vi "Close.vi"(8 "error in (no error)":errorcluster, 11 "SolarShutt in":refnum<class "SolarShutt.lvclass">) -> (0 "error out":errorcluster, 3 "SolarShutt out":refnum<class "SolarShutt.lvclass">)   [LabVIEW 2016]
uses:
  SolarShutt.lvclass
  Controls/Shutter States.ctl
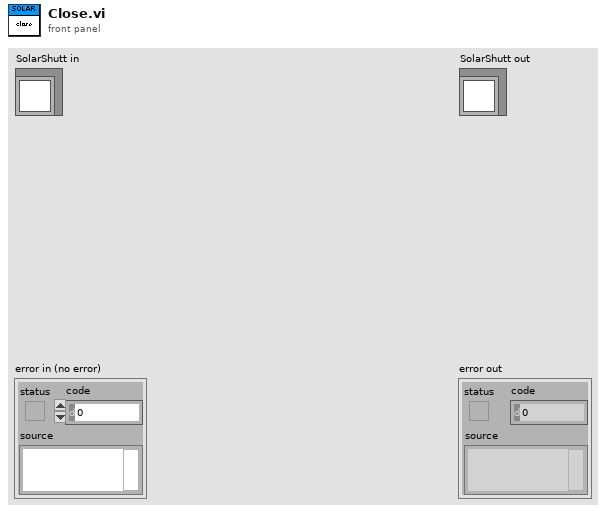
[diagram p1: front panel]
types:
  T1 = typedef "Shutter States.ctl" = enum16{"Open", "Close", "Wait", "Off", "Arm", "Idle"}
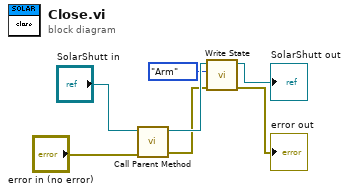
[diagram p0: block diagram]
diagram:
  n1 = call-parent "Call Parent Method"("error in (no error)"="error in (no error)", "UniStableShutter in"="SolarShutt in") -> ("error out"=w3:errorcluster, "UniStableShutter out"=w5:refnum<class "SolarShutt.lvclass">)  [unwired: 8 in]
  n2 = call-dynamic "Write State.vi"("error in (no error)"=w3, "Set"=Shutter_States."Arm", "Shutter in"=w5) -> ("error out"=→"error out":errorcluster, "Shutter out"=→"SolarShutt out":refnum<class "SolarShutt.lvclass">)  [unwired: 7 in]
